vi "Configure Volt Peak.vi"(7 "Channel (1:Channel 1)":i32(ring)=1 items=["Channel 1"=1, "Channel 2"=2], 8 "error in (no error)":errorcluster, 10 "Volt Peak Type (0:Maximum)":i32(ring) items=["Maximum", "Minimum", "Peak-to-Peak", "Average"], 11 "VISA resource name":refnum<visa-resource-name>) -> (0 "error out":errorcluster, 3 "VISA resource name out":refnum<visa-resource-name>)   [LabVIEW 2013, in "Counter.lvlib" / "PICOTEST U62XXA series.lvlib"]
doc: "Configures the settings required for Volt Peak Measurements.\n\n\n<B>Note:</B>\n\nVolt Peak Measurements <B>does not</B> support any <B>post acquisition</B> (Limit, Scale Offset, Statistics) operations. Also, they <B>does not</B> support any <B>Arming</B>."
uses:
  PICOTEST U62XXA series.lvlib
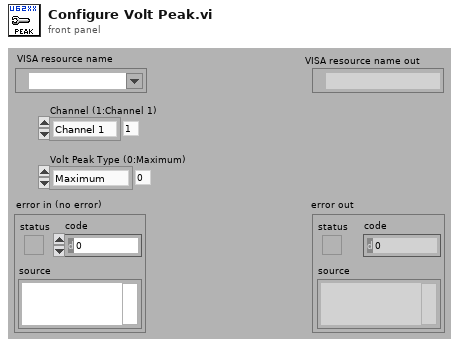
[diagram p1: front panel]
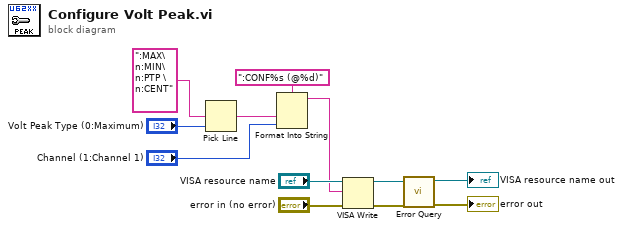
[diagram p0: block diagram]
diagram:
  n1 = Pick Line(multi-line string=":MAX\n:MIN\n:PTP \n:CENT", line index="Volt Peak Type (0:Maximum)") -> (output string=w6:string)  [unwired: 1 in]
  n2 = Format Into String(format string=":CONF%s (@%d)", w6, "Channel (1:Channel 1)") -> (resulting string=w9:string)  [unwired: 2 in, 1 out]
  n3 = VISA Write(VISA resource name="VISA resource name", write buffer=w9, error in (no error)="error in (no error)") -> (VISA resource name out=w5:refnum<visa-resource-name>, error out=w3:errorcluster)  [unwired: 1 out]
  n4 = call "Error Query.vi"("error in (no error)"=w3, "VISA resource name"=w5) -> ("error out"=→"error out":errorcluster, "VISA resource name out"=→"VISA resource name out":refnum<visa-resource-name>)  [unwired: 6 in, 2 out]
